vi "Init Values.vi"(8 "error in (no error)":errorcluster, 11 "ValveControlModule in":refnum<class "ValveControlModule.lvclass">) -> (0 "error out":errorcluster, 3 "ValveControlModule out":refnum<class "ValveControlModule.lvclass">)   [LabVIEW 2020, in "VolatusControl.lvlib" / "ValveControlModule.lvclass"]
uses:
  ValveControlModule.lvclass
  ValveControlModule.lvclass/ValveControlModule.ctl
  lv-vecto/Vecto/Group/Group.lvclass
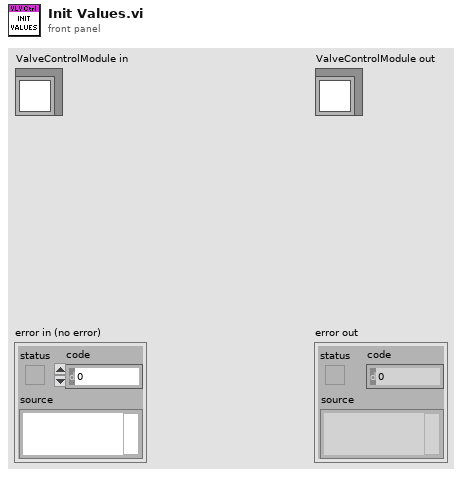
[diagram p1: front panel]
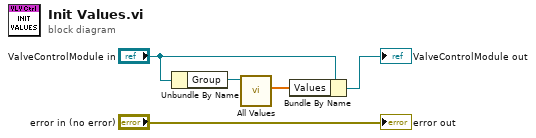
[diagram p0: block diagram]
diagram:
  n1 = Unbundle By Name("ValveControlModule in") -> ("Group"=w3:refnum<class "Group.lvclass">)
  n2 = call "All Values.vi"("Group in"=w3) -> ("Scaled"=w1:dbl[])  [unwired: 6 in, 4 out]
  n3 = Bundle By Name(cluster="ValveControlModule in", "Values"=w1) -> (→"ValveControlModule out":refnum<class "ValveControlModule.lvclass">)
  "error out" <- "error in (no error)"
